vi "TXRefGet.vi"(8 "error in (no error)":errorcluster caption="错误输入（无错误）", 11 "MainPage 输入":refnum<class "MainPage.lvclass">) -> (0 "error out":errorcluster caption="错误输出", 1 "非法引用句柄？":bool, 2 "通讯接口数据":T1, 3 "MainPage 输出":refnum<class "MainPage.lvclass">, 4 "引用":refnum<data-value>)   [LabVIEW 2019, in "MainPage.lvlib" / "MainPage.lvclass"]
uses:
  MainPage.lvclass
  MainPage.lvclass/MainPage.ctl
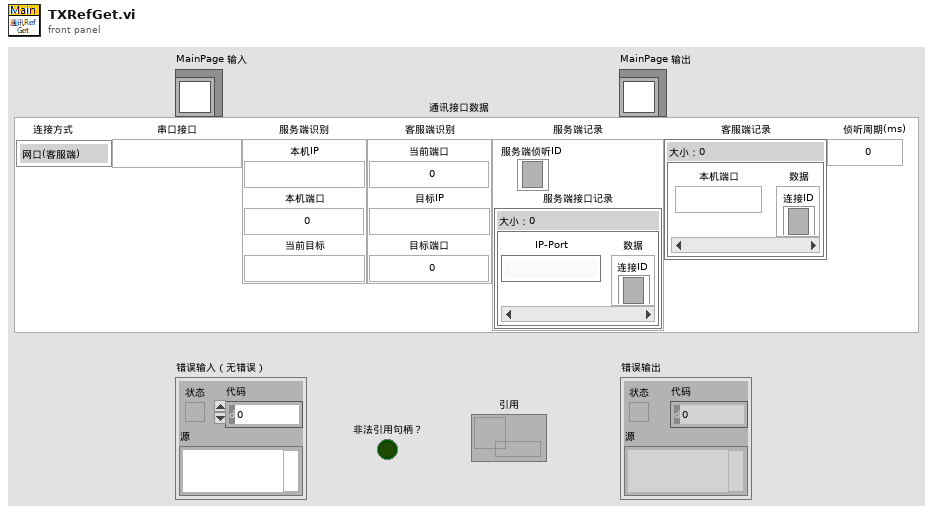
[diagram p1: front panel]
types:
  T1 = typedef "MainPage.lvlib/MainPage.lvclass/DataRef_通讯接口.ctl" = cluster{"连接方式":enum16{"网口(客服端)", "网口(服务端)", "串口"}, "VISA串口名称":refnum<visa-resource-name>, "服务端识别":cluster{"本机IP":string, "本机端口":u16, "当前目标":string}, "客服端识别":cluster{"当前端口":u16, "目标IP":string, "目标端口":u16}, "服务端记录":cluster{"服务端侦听ID":refnum<k5>, "服务端接口记录":map{string, cluster{"连接ID":refnum<k5>}}}, "客服端记录":map{u16, cluster{"连接ID":refnum<k5>}}, "侦听周期(ms)":u32}
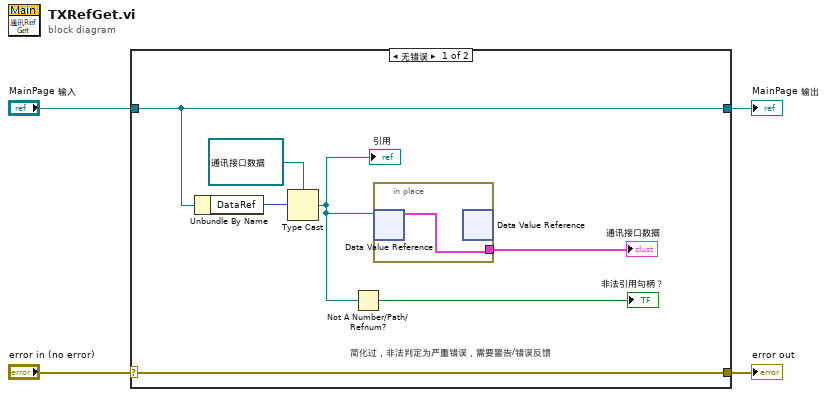
[diagram p0: block diagram]
diagram:
  n1 = case shown="无错误" "error in (no error)" {
    selector: "error in (no error)" -> [w11 w14]
    tunnel: [w11 w14] -> w3
    tunnel: [w10 w13] -> w1
    tunnel: "MainPage 输入" -> [w10 w13]
    frame No Error {
      # "简化过，非法判定为严重错误，需要警告/错误反馈"
      n2 = Unbundle By Name(w10) -> ("DataRef"=w7:u32)
      n3 = Type Cast(type=refnum<data-value> refnum ("通讯接口引用"), x=w7) -> (*(type *) &x=w5:refnum<data-value>)
      "引用" <- w5
      n4 = Not A Number/Path/Refnum?(number/path/refnum=w5) -> (NaN/Path/Refnum?=→"非法引用句柄？":bool)
      n5 = in-place {
        in-place-border: [w12] -> w9
        n6 = in-place-dvr #1(w5) -> (w12:T1)  [unwired: 1 out]
        n7 = in-place-dvr #1() -> ()  [unwired: 1 in, 2 out]
      }
      "通讯接口数据" <- w9
    }
    frame Error {
    }
  }
  "error out" <- w3
  "MainPage 输出" <- w1
